vi "Resizable Panel with Splitter Bars.vi"() -> ()   [LabVIEW 2015]
doc: "This example demonstrates the use of splitter bars to divide the front panel into multiple panes. Each pane can be set up to behave differently depending on the desired function of each pane. In this example the graphical display contained in the lower right pane has the ability to resize with the pane."
panel:
  in  "Load Message":string="Data Loaded"
  in  "Clear Message":string="Data Cleared"
  in  "Stop Message":string="VI Stopped"
  out "Display Message":string
  in  "Stop":bool
  in  "Clear":bool
  in  "Load":bool
  out "Waveform Graph":dynamicdata(graph)
  # "Overview: Demonstrates the use of Splitter Bars to create a resizable panel.\nInstructions:\n1. Run the VI.\n2. Click the Load button to load a Sine waveform into the graph.\n3. Resize the window by dragging its lower right corner. Note that the graph and the string indicator resize with the window.\n4. Click the Clear button to clear the graph.\n5. Click Stop to stop the VI."
  # "Note: The Display Message string and Waveform Graph indicators are set to Scale Object with Pane in their respective right-click menus. This means that when the pane that owns them is resized, the objects will resize with the pane."
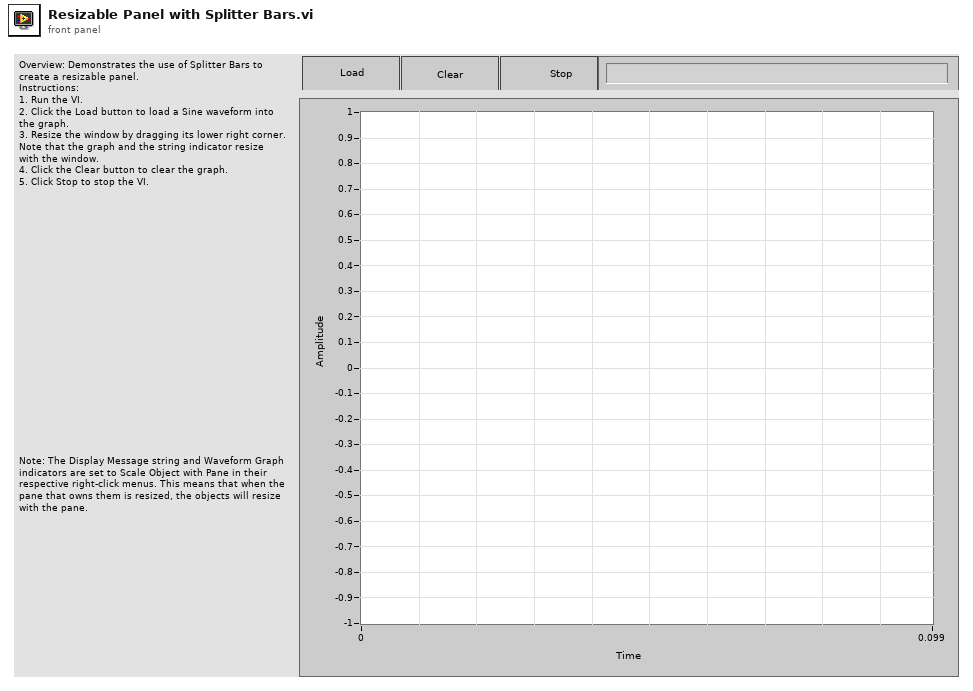
[diagram p1: front panel]
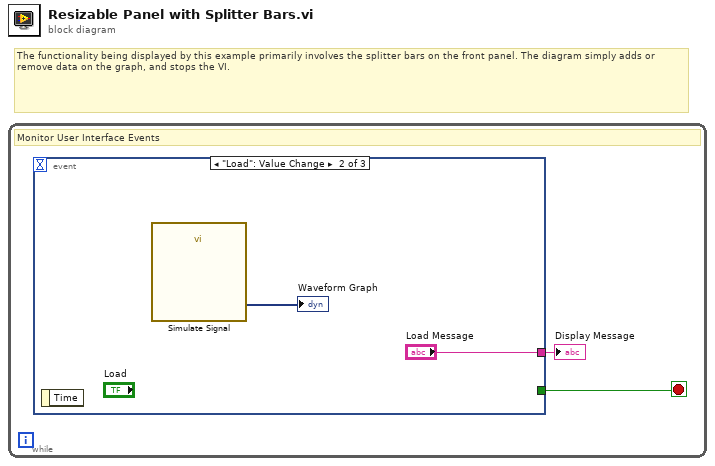
[diagram p0: block diagram]
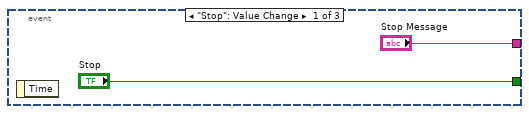
[diagram p2: hidden frame]
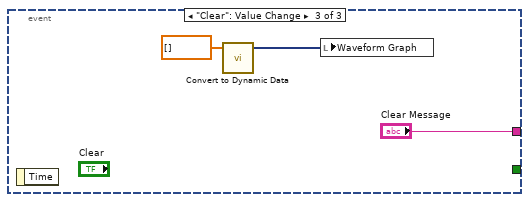
[diagram p3: hidden frame]
diagram:
  # "The functionality being displayed by this example primarily involves the splitter bars on the front panel. The diagram simply adds or remove data on the graph, and stops the VI."
  n1 = while {
    stop <- w2 stop-if-true
    # "Monitor User Interface Events"
    n2 = event shown="[1] \"Load\": Value Change" {
      selector: _ -> [_ _ _]
      dyn-events: _ -> [_ _ _]
      timeout: _ -> [_ _ _]
      tunnel: ["Stop" _ _] -> w2
      tunnel: ["Stop Message" "Load Message" "Clear Message"] -> w1
      event "Stop": Value Change {
        n3 = event-data() -> ()  [unwired: 1 in, 1 out]
      }
      event "Load": Value Change {
        n4 = event-data() -> ()  [unwired: 1 in, 1 out]
        n5 = call "Simulate Signal"() -> ("Sine"=→"Waveform Graph":dynamicdata)  [unwired: 14 in, 1 out]
      }
      event "Clear": Value Change {
        n6 = event-data() -> ()  [unwired: 1 in, 1 out]
        n7 = call "Convert to Dynamic Data"("Array"=dbl[] []) -> ("Dynamic Data Type"=w8:dynamicdata)  [unwired: 3 in]
        n8 = local write "Waveform Graph"(w8) -> ()
      }
    }
    "Display Message" <- w1
  }
